vi "TimerFGV.vi"(10 "Time Target (s)":dbl, 11 "FGV State":T1) -> (2 "Time has Elapsed?":bool, 3 "Elapsed Time (s)":dbl)   [LabVIEW 2019]
uses:
  Controls/FGV_State.ctl
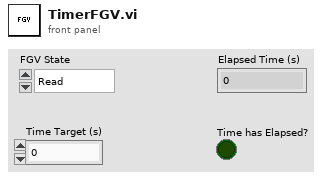
[diagram p1: front panel]
types:
  T1 = typedef "FGV_State.ctl" = enum16{"Read", "Set"}
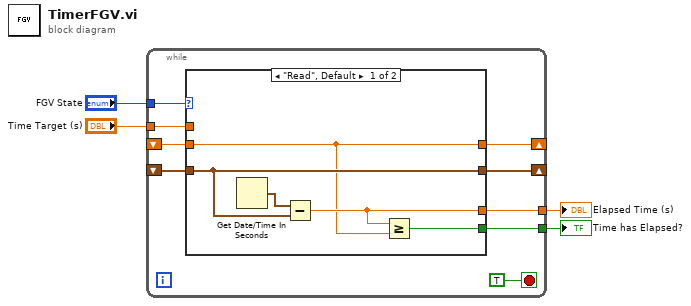
[diagram p0: block diagram]
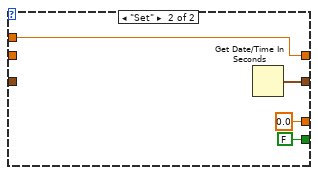
[diagram p2: hidden frame]
diagram:
  n1 = while {
    tunnel: "FGV State" -> [w12]
    shift-right: [w11] -> _
    shift-left: _ -> [w7]
    tunnel: "Time Target (s)" -> [w10]
    shift-right: [w9] -> _
    shift-left: _ -> [w8]
    tunnel: [w6] -> w3
    tunnel: [w5] -> w1
    stop <- TRUE stop-if-true
    n2 = case shown="\"Read\", Default" w12 {
      tunnel: [w17 w22] -> w11
      tunnel: w10 -> [_ w21]
      tunnel: [w15 w21] -> w9
      tunnel: w8 -> [w15 _]
      tunnel: w7 -> [w17 _]
      tunnel: [w16 0.0] -> w6
      tunnel: [w14 FALSE] -> w5
      frame "Read", Default {
        n3 = Get Date/Time In Seconds() -> (seconds since 1Jan1904=w18:timestamp)
        n4 = Subtract(x=w18, y=w17) -> (x-y=w16:dbl)
        n5 = Greater Or Equal?(x=w16, y=w15) -> (x >= y?=w14:bool)
      }
      frame "Set" {
        n6 = Get Date/Time In Seconds() -> (seconds since 1Jan1904=w22:timestamp)
      }
    }
  }
  "Elapsed Time (s)" <- w3
  "Time has Elapsed?" <- w1
